vi "Refresh-available-characteristics.vi"(9 "Temperature value":bool, 10 "Melt-pool charact":bool, 11 "Image characteristics":bool) -> (1 "Unavailable indices":i32[](array[numeric]), 3 "Available":T1[](array[typedef]))   [LabVIEW 2013, in "CameraVision.lvlib" / "CV-Mapping.lvclass"]
uses:
  CV-Mapping.lvclass
  Mapping-characteristic.ctl
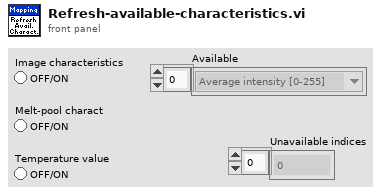
[diagram p1: front panel]
types:
  T1 = typedef "CameraVision.lvlib/CV-Mapping.lvclass/Mapping-characteristic.ctl" = enum16{"Average intensity [0-255]", "Peak intensity [0-255]", "Melt-pool size [mm²]", "Melt-pool aspect ratio []", "Melt-pool fragments []", "Average temperature [°C]", "Max. temperature [°C]", "Min. temperature [°C]", "Std. dev. temperature [°C]"}
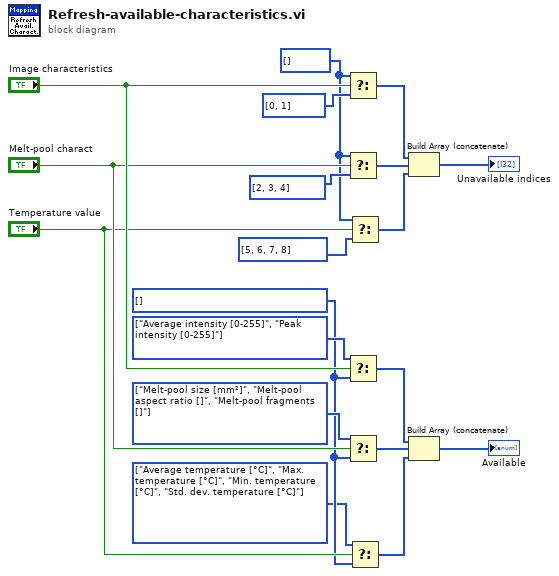
[diagram p0: block diagram]
diagram:
  w2 = T1[] [enum."Average temperature [°C]", enum."Max. temperature [°C]", enum."Min. temperature [°C]", enum."Std. dev. temperature [°C]"] items=["Average intensity [0-255]", "Peak intensity [0-255]", "Melt-pool size [mm²]", "Melt-pool aspect ratio []", "Melt-pool fragments []", "Average temperature [°C]", "Max. temperature [°C]", "Min. temperature [°C]", "Std. dev. temperature [°C]"]
  w3 = T1[] [] items=["Average intensity [0-255]", "Peak intensity [0-255]", "Melt-pool size [mm²]", "Melt-pool aspect ratio []", "Melt-pool fragments []", "Average temperature [°C]", "Max. temperature [°C]", "Min. temperature [°C]", "Std. dev. temperature [°C]"]
  w8 = T1[] [enum."Melt-pool size [mm²]", enum."Melt-pool aspect ratio []", enum."Melt-pool fragments []"] items=["Average intensity [0-255]", "Peak intensity [0-255]", "Melt-pool size [mm²]", "Melt-pool aspect ratio []", "Melt-pool fragments []", "Average temperature [°C]", "Max. temperature [°C]", "Min. temperature [°C]", "Std. dev. temperature [°C]"]
  w9 = T1[] [enum."Average intensity [0-255]", enum."Peak intensity [0-255]"] items=["Average intensity [0-255]", "Peak intensity [0-255]", "Melt-pool size [mm²]", "Melt-pool aspect ratio []", "Melt-pool fragments []", "Average temperature [°C]", "Max. temperature [°C]", "Min. temperature [°C]", "Std. dev. temperature [°C]"]
  w7 = i32[] []
  n1 = Select(t=w7, s="Image characteristics", f=i32[] [0, 1]) -> (s? t:f=w15:i32[])
  n2 = Select(t=w7, s="Melt-pool charact", f=i32[] [2, 3, 4]) -> (s? t:f=w14:i32[])
  n3 = Select(t=w9, s="Image characteristics", f=w3) -> (s? t:f=w5:T1[])
  n4 = Select(t=w8, s="Melt-pool charact", f=w3) -> (s? t:f=w6:T1[])
  n5 = Select(t=w7, s="Temperature value", f=i32[] [5, 6, 7, 8]) -> (s? t:f=w19:i32[])
  n6 = Select(t=w2, s="Temperature value", f=w3) -> (s? t:f=w4:T1[])
  n7 = Build Array (concatenate)(w15, w14, w19) -> (→"Unavailable indices":i32[])
  n8 = Build Array (concatenate)(w5, w6, w4) -> (→"Available":T1[])
